vi "UA to DCAF DataType.vi"(1 "OPC UA Data Type":T1) -> (0 "DCAF Datatype":T2)   [LabVIEW 2013, in "OPC UA configuration.lvclass"]
doc: "Typecast the OPC UA datatype to one compatible with the DCAF engine"
uses:
  OPC UA configuration.lvclass
  <vilib>/NI/Tag Bus/tag/Data Type.ctl
  OPC UA Data Type.ctl
  <vilib>/NI/Tag Bus/tag/tag descriptor.lvclass
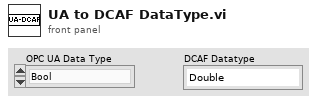
[diagram p1: front panel]
types:
  T1 = typedef "OPC UA configuration.lvclass/OPC UA Data Type.ctl" = enum16{"Bool", "SByte", "Byte", "Int16", "UInt16", "Int32", "UInt32", "Int64", "UInt64", "Float", "Double", "String", "DateTime", "ByteString", "Bool Array", "SByte Array", "Byte Array", "Int16 Array", "UInt16 Array", "Int32 Array", "UInt32 Array", "Int64 Array", "UInt64 Array", "Float Array", "Double Array", "String Array", "DateTime Array", "ByteString Array"}
  T2 = typedef "tag bus.lvlib/tag descriptor.lvclass/Data Type.ctl" = enum16{"Double", "Single", "I64", "I32", "I16", "I8", "U64", "U32", "U16", "U8", "Boolean", "String", "Array of Double", "Array of Single", "Array of I64", "Array of I32", "Array of I16", "Array of I8", "Array of U64", "Array of U32", "Array of U16", "Array of U8", "Array of Boolean", "Array of String"}
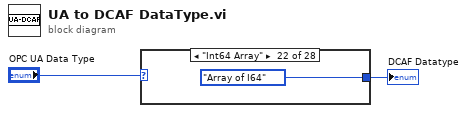
[diagram p0: block diagram]
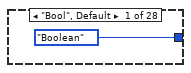
[diagram p2: hidden frame]
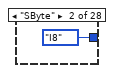
[diagram p3: hidden frame]
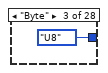
[diagram p4: hidden frame]
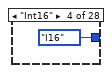
[diagram p5: hidden frame]
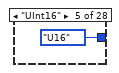
[diagram p6: hidden frame]
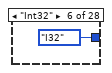
[diagram p7: hidden frame]
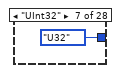
[diagram p8: hidden frame]
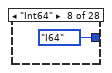
[diagram p9: hidden frame]
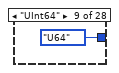
[diagram p10: hidden frame]
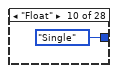
[diagram p11: hidden frame]
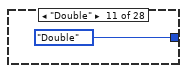
[diagram p12: hidden frame]
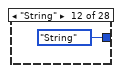
[diagram p13: hidden frame]
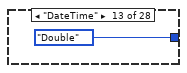
[diagram p14: hidden frame]
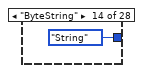
[diagram p15: hidden frame]
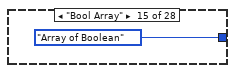
[diagram p16: hidden frame]
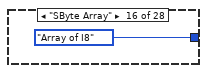
[diagram p17: hidden frame]
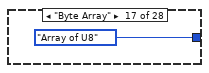
[diagram p18: hidden frame]
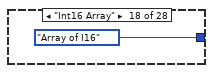
[diagram p19: hidden frame]
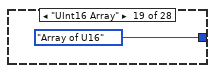
[diagram p20: hidden frame]
diagram:
  n1 = case shown="\"Int64 Array\"" "OPC UA Data Type" {
    tunnel: [Data_Type."Boolean" ("DCAF Datatype") Data_Type."I8" ("DCAF Datatype") Data_Type."U8" ("DCAF Datatype") Data_Type."I16" ("DCAF Datatype") Data_Type."U16" ("DCAF Datatype") Data_Type."I32" ("DCAF Datatype") Data_Type."U32" ("DCAF Datatype") Data_Type."I64" ("DCAF Datatype") Data_Type."U64" ("DCAF Datatype") Data_Type."Single" ("DCAF Datatype") Data_Type."Double" ("DCAF Datatype") Data_Type."String" ("DCAF Datatype") Data_Type."Double" ("DCAF Datatype") Data_Type."String" ("DCAF Datatype") Data_Type."Array of Boolean" ("DCAF Datatype") Data_Type."Array of I8" ("DCAF Datatype") Data_Type."Array of U8" ("DCAF Datatype") Data_Type."Array of I16" ("DCAF Datatype") Data_Type."Array of U16" ("DCAF Datatype") Data_Type."Array of I32" ("DCAF Datatype") Data_Type."Array of U32" ("DCAF Datatype") Data_Type."Array of I64" ("DCAF Datatype") Data_Type."Array of U64" ("DCAF Datatype") Data_Type."Array of Single" ("DCAF Datatype") Data_Type."Array of Double" ("DCAF Datatype") Data_Type."Array of String" ("DCAF Datatype") Data_Type."Array of Double" ("DCAF Datatype") Data_Type."Array of String" ("DCAF Datatype")] -> w2
    frame "Bool", Default {
    }
    frame "SByte" {
    }
    frame "Byte" {
    }
    frame "Int16" {
    }
    frame "UInt16" {
    }
    frame "Int32" {
    }
    frame "UInt32" {
    }
    frame "Int64" {
    }
    frame "UInt64" {
    }
    frame "Float" {
    }
    frame "Double" {
    }
    frame "String" {
    }
    frame "DateTime" {
    }
    frame "ByteString" {
    }
    frame "Bool Array" {
    }
    frame "SByte Array" {
    }
    frame "Byte Array" {
    }
    frame "Int16 Array" {
    }
    frame "UInt16 Array" {
    }
    frame "Int32 Array" {
    }
    frame "UInt32 Array" {
    }
    frame "Int64 Array" {
    }
    frame "UInt64 Array" {
    }
    frame "Float Array" {
    }
    frame "Double Array" {
    }
    frame "String Array" {
    }
    frame "DateTime Array" {
    }
    frame "ByteString Array" {
    }
  }
  "DCAF Datatype" <- w2
